vi "Test DMM.vi"() -> ()   [LabVIEW 2025, in "Aim TTi 1908P DMM.lvlib"]
uses:
  Aim TTi 1908P DMM.lvlib
  Configure.ctl
  72b4c698-04ca-4bd9-a8cd-210e6cdb54c9.vi
  e59d55f9-e56c-48e5-a112-d007c7cd2e68.vi
panel:
  out "error out":errorcluster
  in  "stop":bool
  out "error out 2":errorcluster
  out "Read Measurement":string
  in  "error in":errorcluster
  in  "Adress":string="TCPIP0::192.168.100.10::9221::SOCKET"
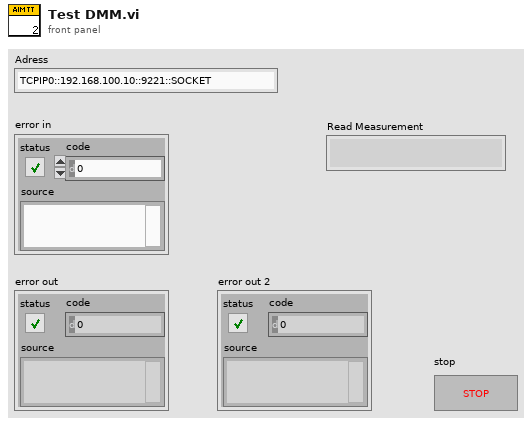
[diagram p1: front panel]
types:
  T1 = typedef "Aim TTi 1908P DMM.lvlib/Configure.ctl" = enum16{"VAC_750V", "VAC_100V", "VDC_AUTO", "VDC_100V", "VDC_1000mV", "VDC_100mV", "VDC_10V", "OHMS_AUTO", "OHMS_10M", "OHMS_10K", "IDC_10A", "IDC_1mA", "IDC_100mA", "IDC_1000mA", "IAC_1mA", "IAC_100mA", "IAC_1000mA", "IAC_10A"}
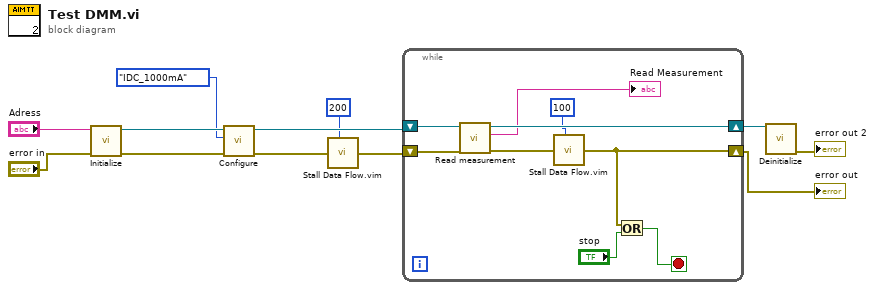
[diagram p0: block diagram]
diagram:
  n1 = call "Initialize.vi"("error in"="error in", "Adress"="Adress") -> ("error out"=w5:errorcluster, "VISA resource name out"=w7:refnum<visa-resource-name>)  [unwired: 6 in]
  n2 = call "Configure.vi"("error in"=w5, "Configuration"=Configure."IDC_1000mA", "VISA resource name"=w7) -> ("error out"=w3:errorcluster, "VISA resource name out"=w6:refnum<visa-resource-name>)  [unwired: 5 in]
  n3 = call "Stall Data Flow.vim"("value in"=w3, "milliseconds to wait"=u32 200) -> ("value out"=w4:errorcluster)  [unwired: 1 out]
  n4 = while {
    shift-right: [w19] -> w10
    shift-left: w6 -> [w20]
    shift-right: [w16] -> w8
    shift-left: w4 -> [w21]
    stop <- w14 stop-if-true
    n5 = call "Read measurement.vi"("error in"=w21, "VISA resource name"=w20) -> ("error out"=w18:errorcluster, "Read data"=→"Read Measurement":string, "VISA resource name out"=w19:refnum<visa-resource-name>)  [unwired: 4 in, 1 out]
    n6 = call "Stall Data Flow.vim"("value in"=w18, "milliseconds to wait"=u32 100) -> ("value out"=w16:errorcluster)  [unwired: 1 out]
    n7 = Or(x=w16, y="stop") -> (x .or. y?=w14:bool)
  }
  "error out" <- w8
  n8 = call "Deinitialize.vi"("VISA resource name"=w10) -> ("error out"=→"error out 2":errorcluster)  [unwired: 8 in]
